vi "Exercise2_week2.vi"() -> ()   [LabVIEW 2015]
panel:
  out "Waveform Chart":dbl(graph)
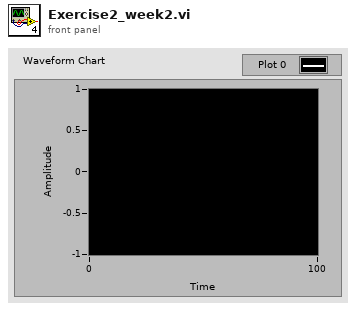
[diagram p1: front panel]
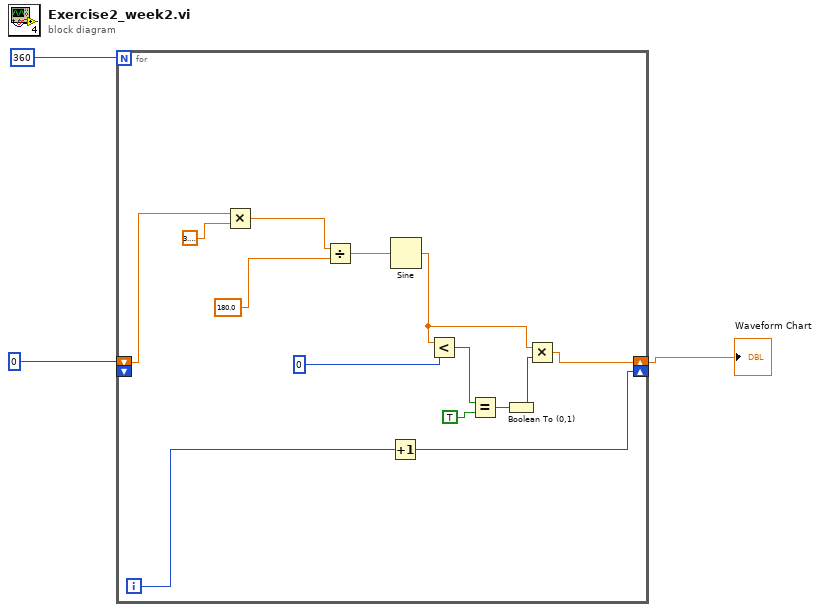
[diagram p0: block diagram]
diagram:
  n1 = for {
    N: 360 -> [_]
    shift-right: [w7] -> w1
    shift-left: 0 -> [w4]
    shift-right: [w5] -> _
    shift-left: _ -> [_]
    i -> [w6]
    n2 = Multiply(x=w4, y=3.141592653589793) -> (x*y=w15:dbl)
    n3 = Divide(x=w15, y=180.0) -> (x/y=w14:dbl)
    n4 = Increment(x=w6) -> (x+1=w5:i32)
    n5 = Sine(x=w14) -> (sin(x)=w8:dbl)
    n6 = Less?(x=w8, y=0) -> (x < y?=w12:bool)
    n7 = Equal?(x=w12, y=TRUE) -> (x = y?=w10:bool)
    n8 = Boolean To (0,1)(Boolean=w10) -> (0, 1=w9:i16)
    n9 = Multiply(x=w8, y=w9) -> (x*y=w7:dbl)
  }
  "Waveform Chart" <- w1
